vi "json Query.vi"   [LabVIEW 2015, in "JSON Document.lvclass"]
uses:
  JSON Document.lvclass
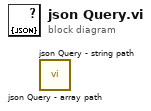
[diagram p0: block diagram]
diagram:
  n1 = call "json Query - array path.vi"() -> ()  [unwired: 8 in, 4 out]
  n2 = call "json Query - string path.vi"() -> ()  [unwired: 8 in, 4 out]
